vi "Config Correct DDNL (OptE).vi"(8 "error in":errorcluster, 10 "DDNL (on)":i32(ring)=1 items=["off", "on"], 11 "VISA resource name":refnum<visa-resource-name>) -> (0 "error out":errorcluster, 3 "VISA resource name out":refnum<visa-resource-name>)   [LabVIEW 2019, in "Andeen-Hagerling 2700(400 firmware).lvlib"]
doc: "Enables or disables Dynamic Differential Non-Linearity.\n\nThis command is only supported on the Option-E version of the AH2700A."
uses:
  Andeen-Hagerling 2700(400 firmware).lvlib
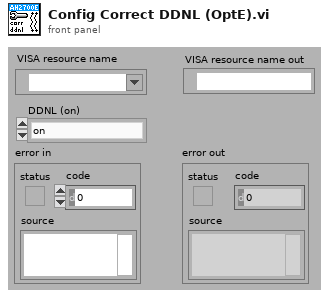
[diagram p1: front panel]
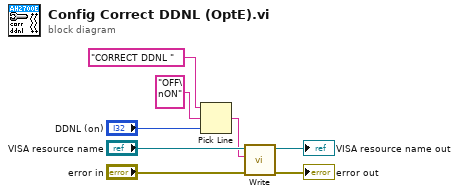
[diagram p0: block diagram]
diagram:
  n1 = Pick Line(string ("")="CORRECT DDNL ", multi-line string="OFF\nON", line index="DDNL (on)") -> (output string=w3:string)
  n2 = call "Write.vi"("error in"="error in", "command"=w3, "VISA resource name"="VISA resource name") -> ("error out"=→"error out":errorcluster, "VISA resource name out"=→"VISA resource name out":refnum<visa-resource-name>)  [unwired: 7 in]
